vi "Stop Panel.vi"(8 "error in (no error)":errorcluster, 10 "SubPanel reference":refnum<vi>, 11 "References in":T1) -> (0 "error out":errorcluster, 2 "SubPanel reference out":refnum<vi>, 3 "References out":T1)   [LabVIEW 2015, in "E2E Tag Exchange editor node.lvclass"]
uses:
  E2E Tag Exchange editor node.lvclass
  references.ctl
  <vilib>/NI/Configuration Framework/Node/StopEvent.ctl
  <vilib>/NI/Configuration Framework/Node/RefreshUIEvent.ctl
  <vilib>/NI/Configuration Framework/Node/CacheState.ctl
  <vilib>/NI/Configuration Framework/Node/NodeChangeEvent.ctl
  <vilib>/NI/Configuration Framework/Node/NodeRef.ctl
  <vilib>/NI/Configuration Framework/Node/NISE_CEF_Node.lvclass
  <vilib>/NI/AMC/Message Queue.ctl
  <vilib>/NI/AMC/Message.ctl
  <vilib>/NI/Tools/Keyed Array/KeyedArray.ctl
  <vilib>/NI/Tools/Keyed Array/Tools_KeyedArray.lvlib
  <vilib>/NI/AMC/AMC.lvlib
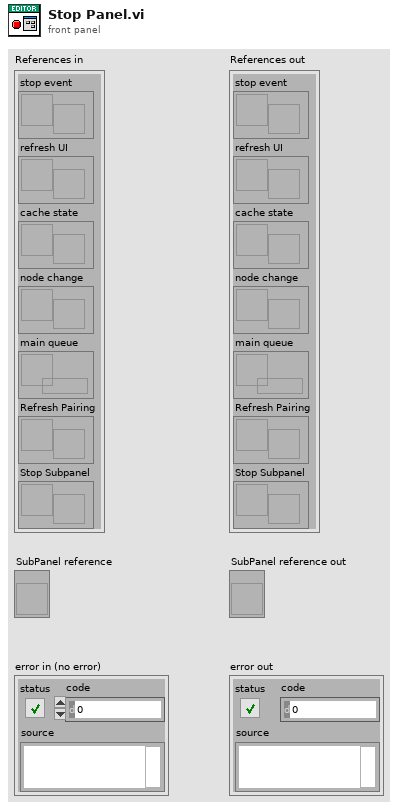
[diagram p1: front panel]
types:
  T1 = typedef "E2E Tag Exchange editor node.lvclass/references.ctl" = cluster{"stop event":T2, "refresh UI":T3, "cache state":T4, "node change":T5, "main queue":T6, "Refresh Pairing":refnum<user-event>, "Stop Subpanel":refnum<user-event>}
  T2 = typedef "NISE_CEF_Node.lvclass/StopEvent.ctl" = refnum<user-event>
  T3 = typedef "NISE_CEF_Node.lvclass/RefreshUIEvent.ctl" = refnum<user-event>
  T4 = typedef "NISE_CEF_Node.lvclass/CacheState.ctl" = refnum<user-event>
  T5 = typedef "NISE_CEF_Node.lvclass/NodeChangeEvent.ctl" = refnum<user-event>
  T6 = typedef "AMC.lvlib/Message Queue.ctl" = refnum<queue>
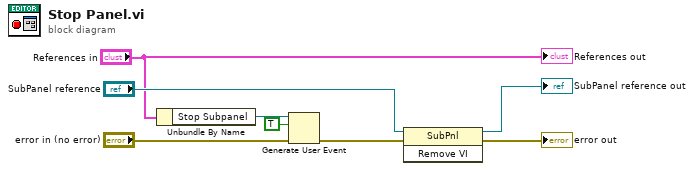
[diagram p0: block diagram]
diagram:
  n1 = Unbundle By Name("References in") -> ("Stop Subpanel"=w1:refnum<user-event>)
  n2 = Generate User Event(user event=w1, event data cluster=TRUE ("event data"), error in="error in (no error)") -> (error out=w6:errorcluster)  [unwired: 1 in, 1 out]
  n3 = invoke class="SubPnl" method="Remove VI"(reference="SubPanel reference", error in=w6) -> (reference out=→"SubPanel reference out":refnum<vi>, error out=→"error out":errorcluster)  [unwired: 1 in, 1 out]
  "References out" <- "References in"
